vi "Configure Self-Alignment Mode.vi"(8 "error in (no error)":errorcluster, 10 "Measurement Mode (IQ)":i32(ring) items=["IQ", "Level", "Verify IQ"], 11 "VISA resource name":refnum<visa-resource-name>) -> (0 "error out":errorcluster, 3 "VISA resource name out":refnum<visa-resource-name>)   [LabVIEW 2015, in "Rohde&Schwarz CMXP Base.lvlib"]
doc: "Selects the measurement mode for self-alignment.\n\nAttribute:\nRSCMXPBASE_ATTR_MEASUREMENT_MODE\n\nRemote-control command:\nCONFigure:BASE:SALignment:MODE"
uses:
  <instrlib>/Rohde&Schwarz CMXP Base/Rohde&Schwarz CMXP Base.lvlib
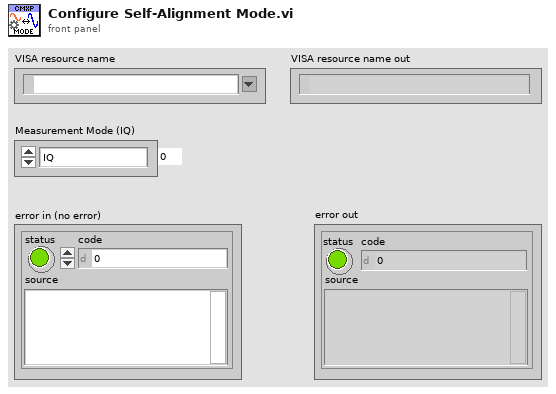
[diagram p1: front panel]
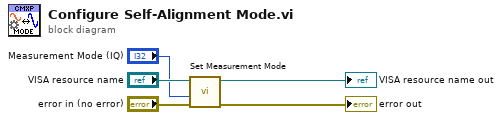
[diagram p0: block diagram]
diagram:
  n1 = call "Set Measurement Mode"("error in (no error)"="error in (no error)", "Measurement Mode (0 - IQ)"="Measurement Mode (IQ)", "instrument handle"="VISA resource name") -> ("error out"=→"error out":errorcluster, "instrument handle out"=→"VISA resource name out":refnum<visa-resource-name>)  [unwired: 7 in]
